vi "Periodic Tasks.vi"(8 "error in":errorcluster) -> (3 "Boolean":bool)   [LabVIEW 2020]
doc: "This VI runs in parallel to other tasks. It can contain as many user-defined periodic loops as you need. These can carry out PID or other sorts of timed response."
uses:
  Systems/Tube Wheel/Tube Wheel_ACT.lvlib
  Systems/Angler/Angler_ACT.lvlib
  Systems/SwerveDrive/SwerveDrive_ACT_ts.lvlib
  Systems/Game Controller/GameController_SEN.lvlib
  Systems/PigeonIMU/PigeonIMU_SEN_ts.lvlib
  Systems/Feeder/Feeder_ACT.lvlib
  Systems/Shooter/Shooter_ACT.lvlib
  Systems/NTV Read Write/NTV Read Write.lvlib
  Systems/SwerveDrive AM/Swerve AM_ACT.lvlib
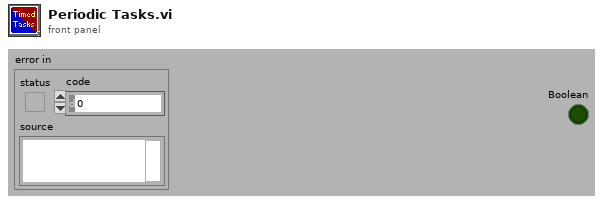
[diagram p1: front panel]
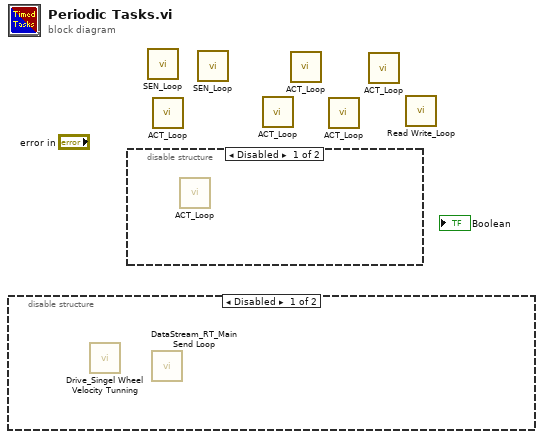
[diagram p0: block diagram]
diagram:
  n1 = disable-structure shown="Disabled" {
    frame Disabled {
      n2 = call "Drive_Singel Wheel Velocity Tunning.vi"() -> ()  [unwired: 12 in]
      n3 = call "DataStream_RT_Main Send Loop.vi"() -> ()  [unwired: 12 in]
    }
    frame Enabled {
    }
  }
  n4 = disable-structure shown="Disabled" {
    frame Disabled {
      n5 = call "ACT_Loop.vi"() -> ()  [unwired: 12 in]
    }
    frame Enabled {
    }
  }
  n6 = call "SEN_Loop.vi"() -> ()  [unwired: 12 in]
  n7 = call "ACT_Loop.vi"() -> ()  [unwired: 12 in]
  n8 = call "SEN_Loop.vi"() -> ()  [unwired: 12 in]
  n9 = call "ACT_Loop.vi"() -> ()  [unwired: 12 in]
  n10 = call "ACT_Loop.vi"() -> ()  [unwired: 12 in]
  n11 = call "ACT_Loop.vi"() -> ()  [unwired: 12 in]
  n12 = call "ACT_Loop.vi"() -> ()  [unwired: 12 in]
  n13 = call "Read Write_Loop.vi"() -> ()  [unwired: 12 in]
